vi "Each_Refdata&Ref_monitordata_struct_Add.vi"(6 "Active Sensors":bool[](array[boolean]), 7 "Ref_monitordata_struct输入":refnum<k24>[](array[refnum]), 8 "错误输入（无错误）":errorcluster, 9 "Controls[]":refnum<vi>[](array[refnum]), 10 "Refdata_struct输入":refnum<k24>[](array[refnum])) -> (0 "错误输出":errorcluster, 1 "Refdata_struct输出":refnum<k24>[](array[refnum]), 2 "Ref_monitordata_struct输出":refnum<k24>[](array[refnum]))   [LabVIEW 2017]
doc: "for reference power data & reference monitor data"
uses:
  D:/test/PDLSTS/LV_PDL LvVer17.0/LV_PDL_x64/DLL/STSProcess.dll
  DLL/STSProcess.dll
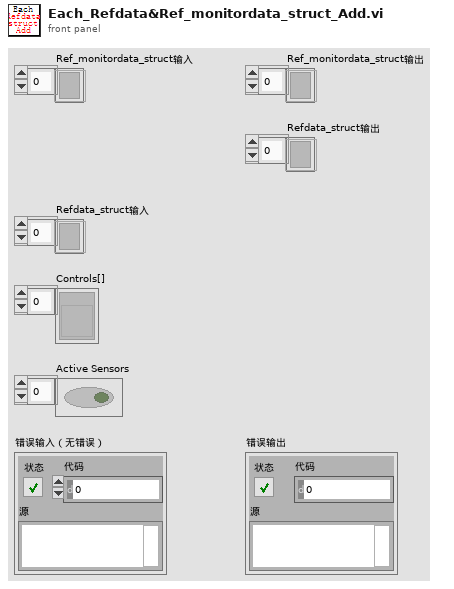
[diagram p1: front panel]
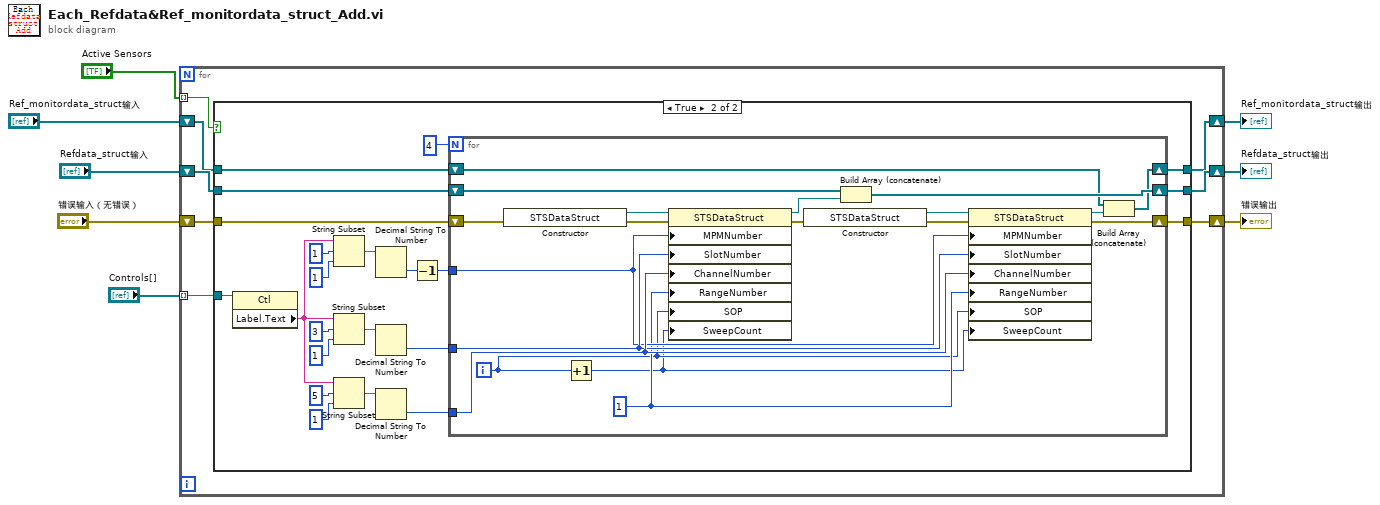
[diagram p0: block diagram]
diagram:
  n1 = for {
    tunnel: "Controls[]" -> [w15] mode=indexing
    tunnel: "Active Sensors" -> [w16] mode=indexing
    shift-right: [w13] -> w6
    shift-left: "Refdata_struct输入" -> [w14]
    shift-right: [w11] -> w5
    shift-left: "Ref_monitordata_struct输入" -> [w12]
    shift-right: [w9] -> w8
    shift-left: "错误输入（无错误）" -> [w10]
    n2 = case shown="True" w16 {
      tunnel: w15 -> [_ w31]
      tunnel: w14 -> [w18 w20]
      tunnel: [w18 w26] -> w13
      tunnel: w12 -> [w19 w25]
      tunnel: [w19 w24] -> w11
      tunnel: w10 -> [w17 w23]
      tunnel: [w17 w22] -> w9
      frame False {
      }
      frame True {
        n3 = property class="Ctl"(reference=w31) -> ("Label.Text"=w30:string)  [unwired: 1 in, 2 out]
        n4 = String Subset(string=w30, offset (0)=1 ("偏移量(0)"), length (rest)=1 ("长度（剩余）")) -> (substring=w34:string)
        n5 = String Subset(string=w30, offset (0)=3 ("偏移量(0)"), length (rest)=1 ("长度（剩余）")) -> (substring=w35:string)
        n6 = String Subset(string=w30, offset (0)=5 ("偏移量(0)"), length (rest)=1 ("长度（剩余）")) -> (substring=w33:string)
        n7 = Decimal String To Number(string=w34) -> (number=w32:i32)  [unwired: 2 in, 1 out]
        n8 = Decimal String To Number(string=w35) -> (number=w28:i32)  [unwired: 2 in, 1 out]
        n9 = Decimal String To Number(string=w33) -> (number=w29:i32)  [unwired: 2 in, 1 out]
        n10 = Decrement(x=w32) -> (x-1=w27:i32)
        n11 = for {
          N: 4 -> [_]
          tunnel: w29 -> [w58]
          tunnel: w28 -> [w57]
          tunnel: w27 -> [w56]
          shift-right: [w48] -> w22
          shift-left: w23 -> [w49]
          shift-right: [w50] -> w24
          shift-left: w25 -> [w52]
          shift-right: [w53] -> w26
          shift-left: w20 -> [w45]
          i -> [w43]
          w44 = 1 ("RangeNumber")
          n12 = constructor class="STSDataStruct"(error in=w49) -> (reference out=w46:refnum<k24>, error out=w47:errorcluster)  [unwired: 2 in, 1 out]
          n13 = Increment(x=w43) -> (x+1=w42:i32)
          n14 = property class="STSDataStruct"(reference=w46, error in=w47, "MPMNumber"=w56, "SlotNumber"=w57, "ChannelNumber"=w58, "RangeNumber"=w44, "SOP"=w43, "SweepCount"=w42) -> (reference out=w54:refnum<k24>, error out=w55:errorcluster)
          n15 = constructor class="STSDataStruct"(error in=w55) -> (reference out=w60:refnum<k24>, error out=w59:errorcluster)  [unwired: 2 in, 1 out]
          n16 = Build Array (concatenate)(w45, w54) -> (w53:refnum<k24>[])
          n17 = property class="STSDataStruct"(reference=w60, error in=w59, "MPMNumber"=w56, "SlotNumber"=w57, "ChannelNumber"=w58, "RangeNumber"=w44, "SOP"=w43, "SweepCount"=w42) -> (reference out=w51:refnum<k24>, error out=w48:errorcluster)
          n18 = Build Array (concatenate)(w52, w51) -> (w50:refnum<k24>[])
        }
      }
    }
  }
  "错误输出" <- w8
  "Refdata_struct输出" <- w6
  "Ref_monitordata_struct输出" <- w5
